vi "Cluster.vi"() -> ()   [LabVIEW 2016]
panel:
  out "簇2":T1
  in  "簇1":T1
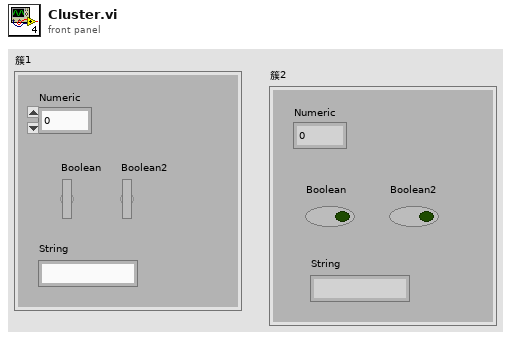
[diagram p1: front panel]
types:
  T1 = cluster{"Numeric":dbl, "Boolean":bool, "Boolean2":bool, "String":string}
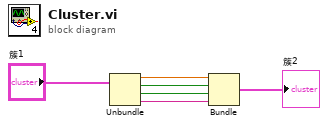
[diagram p0: block diagram]
diagram:
  n1 = Unbundle("簇1") -> ("Numeric"=w4:dbl, "Boolean"=w3:bool, "Boolean2"=w2:bool, "String"=w1:string)
  n2 = Bundle("Numeric"=w4, "Boolean"=w3, "Boolean2"=w2, "String"=w1) -> (→"簇2":T1)  [unwired: 1 in]
